vi "Add_to_speed_calib_file.vi"(2 "Desired Velocity":dbl format="%.2f", 3 "Max Velocity":dbl format="%.2f", 4 "New Row":dbl[](array[numeric]) format="%.2f", 5 "Tunnel Heated?":bool, 6 "Rig Name":string, 7 "Mode":enum16{"Add Row", "Get Error Value"}(ring)) -> (0 "Tweaked Demand":dbl format="%.4f", 1 "Calib Tweak %":dbl format="%.4f")   [LabVIEW 2010]
uses:
  Anemometry/Anemometry Sub Vis/File/Setup_Filetype.ctl
  Anemometry/Anemometry Sub Vis/Controls/In_Range.ctl
panel:
  out "Array":dbl[][](array[numeric]) format="%.4f"
  out "Channel Values":string[][](array[string])
  # "Dem Vel       Calib Tweak   Meas Vel"
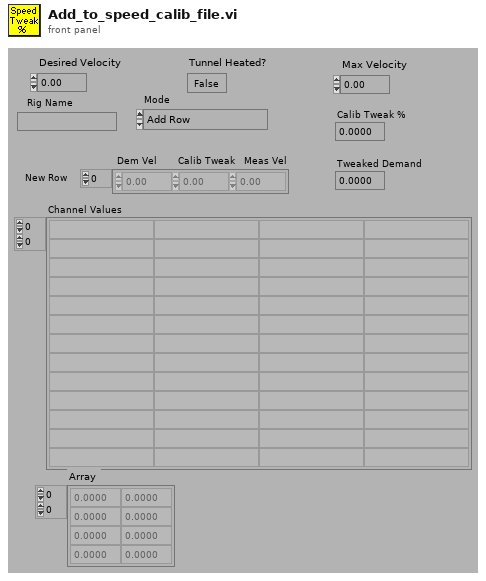
[diagram p1: front panel]
types:
  T1 = typedef "Setup_Filetype.ctl" = enum16{"Measurement Setups", "Calibration Setups", "General", "Results File Plotter Setups", "Speed Calib Tweaks"}
  T2 = typedef "In_Range.ctl" = enum16{"%", "±", "% & ±"}
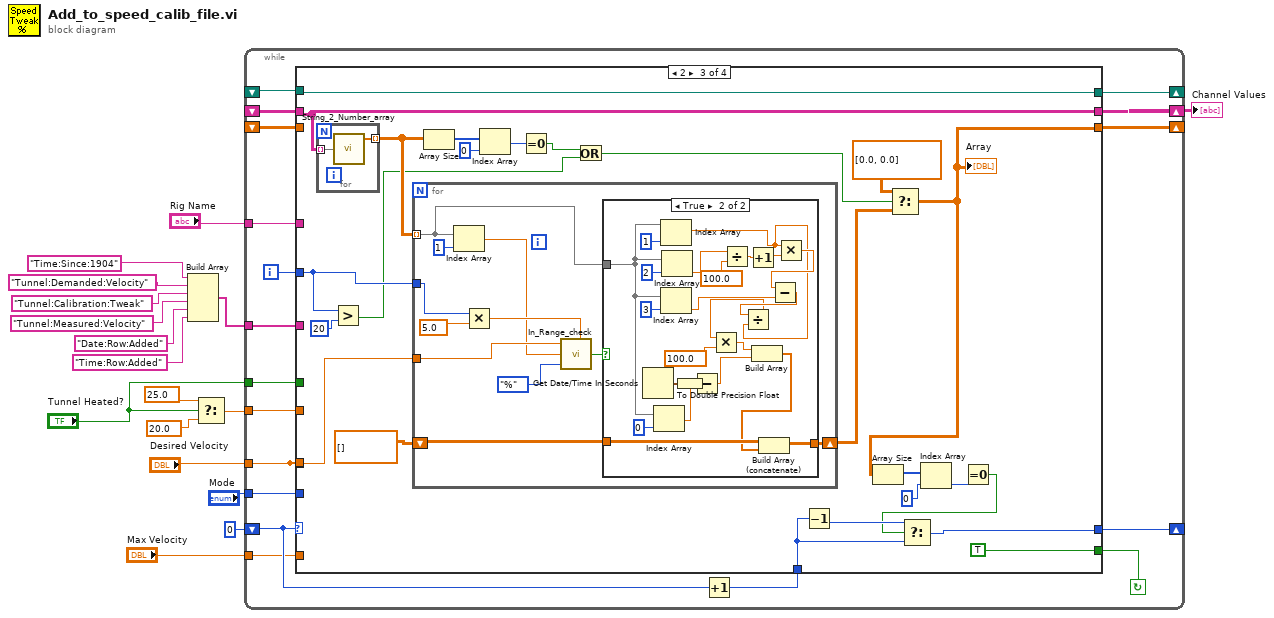
[diagram p0: block diagram]
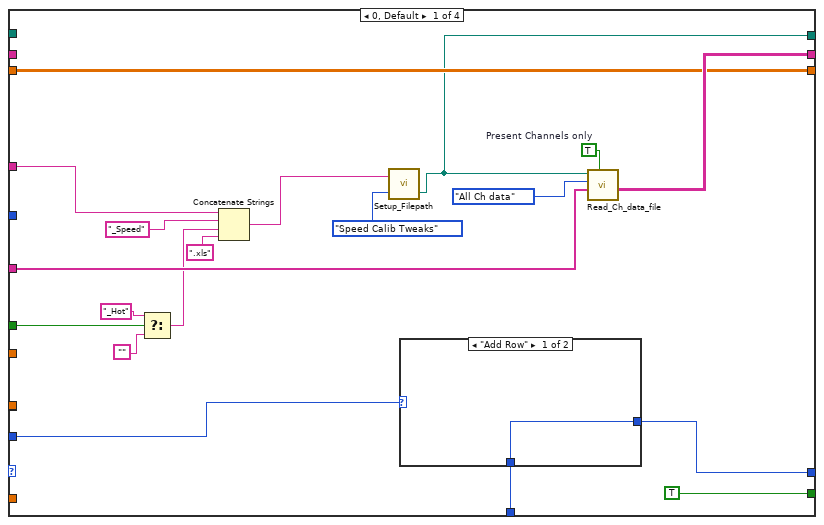
[diagram p2: hidden frame]
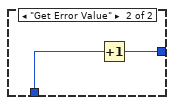
[diagram p3: hidden frame]
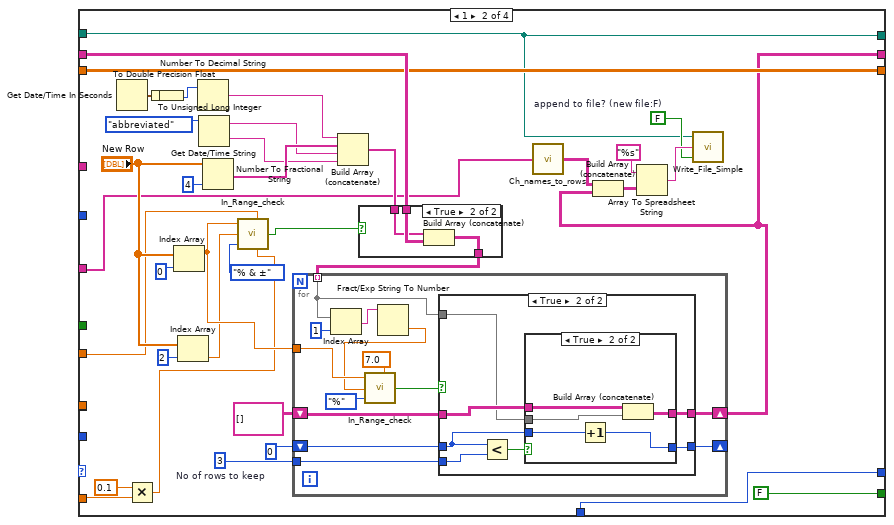
[diagram p4: hidden frame]
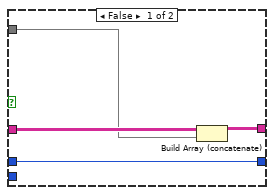
[diagram p6: hidden frame]
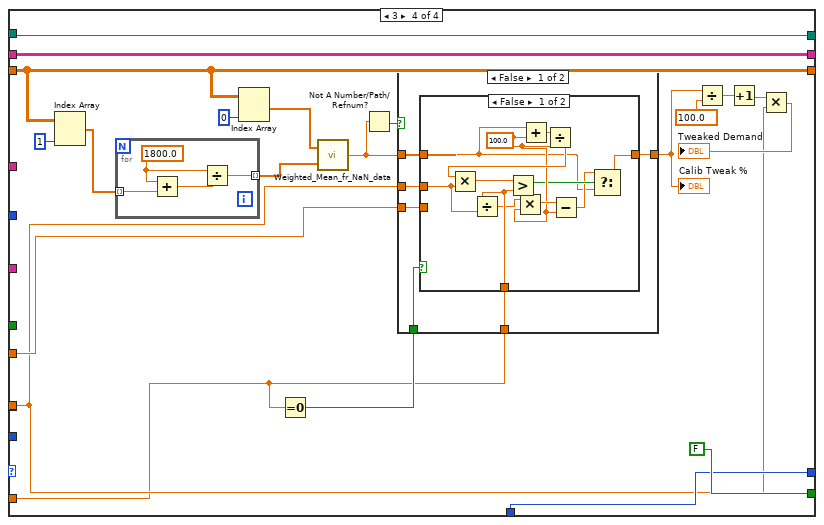
[diagram p9: hidden frame]
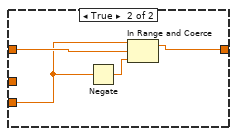
[diagram p10: hidden frame]
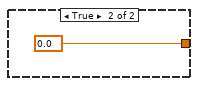
[diagram p11: hidden frame]
diagram:
  n1 = Build Array("Time:Since:1904" ("Substring"), "Tunnel:Demanded:Velocity" ("Substring"), "Tunnel:Calibration:Tweak" ("Substring"), "Tunnel:Measured:Velocity" ("Substring"), "Date:Row:Added" ("Substring"), "Time:Row:Added" ("Substring")) -> (w12:string[])
  n2 = Select(t=25.0 ("Min"), s="Tunnel Heated?", f=20.0 ("Max")) -> (s? t:f=w6:dbl)
  n3 = while {
    tunnel: w6 -> [w19]
    tunnel: "Desired Velocity" -> [w20]
    tunnel: "Tunnel Heated?" -> [w21]
    tunnel: "Rig Name" -> [w22]
    shift-left: _ -> [w23]
    shift-right: [w24] -> _
    tunnel: w12 -> [w30]
    shift-left: _ -> [w27]
    shift-right: [w28] -> w11
    shift-left: _ -> [w26]
    shift-right: [w29] -> _
    tunnel: "Mode" -> [w33]
    shift-left: 0 -> [w34]
    shift-right: [w32] -> _
    tunnel: "Max Velocity" -> [w18]
    i -> [w25]
    stop <- w35 continue-if-true
    n4 = Increment(x=w34) -> (x+1=w31:i32)
    n5 = case shown="2" w34 {
      tunnel: [TRUE FALSE TRUE FALSE] -> w35
      tunnel: w33 -> [w52 _ _ _]
      tunnel: [w51 w84 w150 w206] -> w32
      tunnel: w31 -> [w50 w84 w152 w206]
      tunnel: w30 -> [w49 w63 _ _]
      tunnel: [w36 w64 w149 w211] -> w29
      tunnel: [w48 w62 w148 w210] -> w28
      tunnel: w27 -> [_ w90 w148 w210]
      tunnel: w26 -> [_ w64 w149 w211]
      tunnel: w25 -> [_ _ w137 _]
      tunnel: [w45 w88 w131 w194] -> w24
      tunnel: w23 -> [w45 w88 _ w194]
      tunnel: w22 -> [w44 _ _ _]
      tunnel: w21 -> [w40 _ _ _]
      tunnel: w20 -> [_ _ w141 _]
      tunnel: w20 -> [_ _ _ w193]
      tunnel: w19 -> [_ w58 _ w200]
      tunnel: w18 -> [_ w61 _ w191]
      frame 0, Default {
        w47 = TRUE  # Present Channels only
        n6 = Select(t="_Hot", s=w40, f="") -> (s? t:f=w41:string)
        n7 = Concatenate Strings(w44, "_Speed" ("Substring"), w41, ".xls" ("string")) -> (w37:string)
        n8 = call "Setup_Filepath.vi"("Setup File Type"=Setup_Filetype."Speed Calib Tweaks", "Filename in"=w37) -> ("Filename Out"=w36:path)  [unwired: 1 out]
        n9 = case shown="\"Add Row\"" w52 {
          tunnel: [w55 w56] -> w51
          tunnel: w50 -> [w55 w57]
          frame "Add Row" {
          }
          frame "Get Error Value" {
            n10 = Increment(x=w57) -> (x+1=w56:i32)
          }
        }
        n11 = call "Read_Ch_data_file.vi"("Present Channels only"=w47, "Present Channels"=w49, "Output"=enum16{"All Ch data", "The last few rows"}."All Ch data", "Filename"=w36) -> ("Channel Values"=w48:string[][])  [unwired: 1 in, 4 out]
      }
      frame 1 {
        w65 = FALSE  # append to file? (new file:F)
        w82 = 3  # No of rows to keep
        n12 = Get Date/Time In Seconds() -> (seconds since 1Jan1904=w76:timestamp)
        n13 = Multiply(x=0.1, y=w61) -> (x*y=w59:dbl)
        n14 = To Double Precision Float(number=w76) -> (double precision float=w92:dbl)
        n15 = To Unsigned Long Integer(number=w92) -> (unsigned 32bit integer=w81:u32)
        n16 = Index Array(array="New Row", index=0 ("Index")) -> (element=w73:dbl)
        n17 = Index Array(array="New Row", index=2 ("Index")) -> (element=w72:dbl)
        n18 = Number To Decimal String(number=w81) -> (decimal integer string=w91:string)  [unwired: 1 out]
        n19 = Get Date/Time String(date format (0)=enum16{"short", "long", "abbreviated"}."abbreviated") -> (date string=w79:string, time string=w78:string)  [unwired: 2 out]
        n20 = Number To Fractional String(number="New Row", precision (6)=i16 4) -> (F-format string=w87:string[])  [unwired: 2 out]
        n21 = call "In_Range_check.vi"("±"=w59, "%"=w58, "Mode"=In_Range."% & ±", "Value"=w72, "Setpoint"=w73) -> ("In Range"=w70:bool)  [unwired: 2 out]
        n22 = Build Array (concatenate)(w91, w87, w79, w78) -> (w89:string[])
        n23 = case shown="True" w70 {
          tunnel: w90 -> [w95 w98]
          tunnel: w89 -> [_ w97]
          tunnel: [w95 w96] -> w86
          frame False {
          }
          frame True {
            n24 = Build Array (concatenate)(w97, w98) -> (w96:string[][])
          }
        }
        n25 = for {
          tunnel: w73 -> [w110]
          tunnel: w86 -> [w104] mode=indexing
          shift-right: [w102] -> w62
          shift-left: string[][] [] -> [w103]
          shift-right: [w101] -> _
          shift-left: 0 -> [w100]
          tunnel: w82 -> [w99]
          n26 = Index Array(array=w104, index=1 ("Index")) -> (element=w108:string)
          n27 = Fract/Exp String To Number(string=w108) -> (number=w107:dbl)  [unwired: 4 out]
          n28 = call "In_Range_check.vi"("%"=7.0, "Mode"=In_Range."%", "Value"=w107, "Setpoint"=w110) -> ("In Range"=w105:bool)  [unwired: 1 in, 2 out]
          n29 = case shown="True" w105 {
            tunnel: w104 -> [w114 w120]
            tunnel: w103 -> [w115 w121]
            tunnel: [w113 w119] -> w102
            tunnel: [w112 w117] -> w101
            tunnel: w100 -> [w112 w118]
            tunnel: w99 -> [_ w116]
            frame False {
              n30 = Build Array (concatenate)(w115, w114) -> (w113:string[][])
            }
            frame True {
              n31 = Less?(x=w118, y=w116) -> (x < y?=w122:bool)
              n32 = case shown="True" w122 {
                tunnel: w121 -> [w124 w129]
                tunnel: w120 -> [_ w128]
                tunnel: [w124 w127] -> w119
                tunnel: w118 -> [w123 w126]
                tunnel: [w123 w125] -> w117
                frame False {
                }
                frame True {
                  n33 = Increment(x=w126) -> (x+1=w125:i32)
                  n34 = Build Array (concatenate)(w129, w128) -> (w127:string[][])
                }
              }
            }
          }
        }
        n35 = call "Ch_names_to_rows.vi"("Channel Names"=w63) -> ("3 Row names"=w69:string[][])
        n36 = Build Array (concatenate)(w69, w62) -> (w67:string[][])
        n37 = Array To Spreadsheet String(array=w67, 3:"%s" ("format string")) -> (spreadsheet string=w66:string)  [unwired: 1 out]
        n38 = call "Write_File_Simple.vi"("append to file? (new file:F)"=w65, "character string"=w66, "file path"=w64) -> ()  [unwired: 2 out]
      }
      frame 2 {
        n39 = for {
          tunnel: w148 -> [w155] mode=indexing
          tunnel: [w154] -> w145 mode=indexing
          n40 = call "String_2_Number_array.vi"("Input String"=w155) -> ("Values"=w154:dbl[])
        }
        n41 = Greater?(x=w137, y=20) -> (0:w133:bool)
        n42 = for {
          tunnel: w145 -> [w160] mode=indexing
          tunnel: w137 -> [w157]
          tunnel: w141 -> [w165]
          shift-right: [w159] -> w132
          shift-left: dbl[][] [] -> [w161]
          n43 = Index Array(array=w160, index=1 ("Index")) -> (element=w156:dbl)
          n44 = Multiply(x=w157, y=5.0 ("x")) -> (x*y=w163:dbl)
          n45 = call "In_Range_check.vi"("%"=w163, "Mode"=In_Range."%", "Value"=w156, "Setpoint"=w165) -> ("In Range"=w162:bool)  [unwired: 1 in, 2 out]
          n46 = case shown="True" w162 {
            tunnel: w161 -> [w167 w190]
            tunnel: w160 -> [_ w176]
            tunnel: [w167 w189] -> w159
            frame False {
            }
            frame True {
              n47 = Get Date/Time In Seconds() -> (seconds since 1Jan1904=w174:timestamp)
              n48 = Index Array(array=w176, index=0 ("Index")) -> (element=w185:dbl)
              n49 = Index Array(array=w176, index=1 ("Index")) -> (element=w170:dbl)
              n50 = Index Array(array=w176, index=3 ("Index")) -> (element=w172:dbl)
              n51 = Index Array(array=w176, index=2 ("Index")) -> (element=w179:dbl)
              n52 = To Double Precision Float(number=w174) -> (double precision float=w186:dbl)
              n53 = Subtract(x=w186, y=w185) -> (x-y=w184:dbl)
              n54 = Divide(x=w179, y=100.0) -> (x/y=w180:dbl)
              n55 = Increment(x=w180) -> (x+1=w178:dbl)
              n56 = Multiply(x=w170, y=w178) -> (x*y=w173:dbl)
              n57 = Subtract(x=w173, y=w172) -> (x-y=w171:dbl)
              n58 = Divide(x=w171, y=w170) -> (x/y=w168:dbl)
              n59 = Multiply(x=w168, y=100.0) -> (x*y=w169:dbl)
              n60 = Build Array(w169, w184) -> (w183:dbl[])
              n61 = Build Array (concatenate)(w190, w183) -> (w189:dbl[][])
            }
          }
        }
        n62 = Array Size(array=w145) -> (size(s)=w144:i32[])
        n63 = Index Array(array=w144, index=0 ("Index")) -> (element=w142:i32)
        n64 = Equal To 0?(x=w142) -> (x = 0?=w135:bool)
        n65 = Or(x=w135, y=w133) -> (x .or. y?=w134:bool)
        n66 = Decrement(x=w152) -> (x-1=w151:i32)
        n67 = Select(t=dbl[][] [[0.0, 0.0]], s=w134, f=w132) -> (s? t:f=w131:dbl[][])
        "Array" <- w131
        n68 = Array Size(array=w131) -> (size(s)=w140:i32[])
        n69 = Index Array(array=w140, index=0 ("Index")) -> (element=w139:i32)
        n70 = Equal To 0?(x=w139) -> (x = 0?=w130:bool)
        n71 = Select(t=w151, s=w130, f=w152) -> (s? t:f=w150:i32)
      }
      frame 3 {
        n72 = Index Array(array=w194, index (col)=1 ("Index")) -> (element=w202:dbl[])  [unwired: 1 in]
        n73 = for {
          tunnel: w202 -> [w215] mode=indexing
          tunnel: [w212] -> w201 mode=indexing
          w213 = 1800.0
          n74 = Add(x=w213, y=w215) -> (x+y=w214:dbl)
          n75 = Divide(x=w213, y=w214) -> (x/y=w212:dbl)
        }
        n76 = Index Array(array=w194, index (col)=0 ("Index")) -> (element=w203:dbl[])  [unwired: 1 in]
        n77 = Equal To 0?(x=w191) -> (x = 0?=w192:bool)
        n78 = call "Weighted_Mean_fr_NaN_data.vi"("Weighting"=w201, "Data"=w203) -> ("Mean value"=w207:dbl)
        n79 = Not A Number/Path/Refnum?(number/path/refnum=w207) -> (NaN/Path/Refnum?=w208:bool)
        n80 = case shown="False" w208 {
          tunnel: w207 -> [w219 _]
          tunnel: [w218 0.0 ("Clamped output")] -> w199
          tunnel: w200 -> [w216 _]
          tunnel: w193 -> [w221 _]
          tunnel: w191 -> [w220 _]
          tunnel: w192 -> [w217 _]
          frame False {
            n81 = case shown="False" w217 {
              tunnel: w221 -> [w230 _]
              tunnel: w220 -> [w229 _]
              tunnel: w219 -> [w223 w237]
              tunnel: [w222 w234] -> w218
              tunnel: w216 -> [_ w236]
              frame False {
                w226 = 100.0 ("y")
                n82 = Divide(x=w229, y=w230) -> (x/y=w228:dbl)
                n83 = Multiply(x=w228, y=w226) -> (x*y=w227:dbl)
                n84 = Add(x=w223, y=w226) -> (x+y=w233:dbl)
                n85 = Divide(x=w233, y=w226) -> (x/y=w232:dbl)
                n86 = Multiply(x=w232, y=w230) -> (x*y=w231:dbl)
                n87 = Greater?(x=w231, y=w229) -> (0:w225:bool)
                n88 = Subtract(x=w227, y=w226) -> (x-y=w224:dbl)
                n89 = Select(t=w224, s=w225, f=w223) -> (s? t:f=w222:dbl)
              }
              frame True {
                n90 = Negate(x=w236) -> (-x=w235:dbl)
                n91 = In Range and Coerce(upper limit=w236, x=w237, lower limit=w235) -> (coerced(x)=w234:dbl)  [unwired: 1 out]
              }
            }
          }
          frame True {
          }
        }
        "Calib Tweak %" <- w199
        n92 = Divide(x=w199, y=100.0) -> (x/y=w197:dbl)
        n93 = Increment(x=w197) -> (x+1=w196:dbl)
        n94 = Multiply(x=w196, y=w193) -> (x*y=→"Tweaked Demand":dbl)
      }
    }
  }
  "Channel Values" <- w11
